vi "Import Asset Configuration.vi"(6 "Asset Configuration File":path, 8 "error in (no error)":errorcluster, 11 "InsightCM Console Wrapper in":refnum<class "InsightCM Console Wrapper.lvclass">) -> (0 "error out":errorcluster, 3 "InsightCM Console Wrapper out":refnum<class "InsightCM Console Wrapper.lvclass">)   [LabVIEW 2020, in "InsightCM Console Wrapper.lvclass"]
doc: "Imports asset configuration to the server using an Excel File (*.xlsx) exported form the same or another server.\n\nConsole command -> importassetspreadsheet -f [filepath]"
uses:
  InsightCM Console Wrapper.lvclass
  C:/Users/fflores/Documents/GitHub Projects/LabVIEW-CLI-Wrapper/Console Wrapper/Console Wrapper.lvclass
  Console Wrapper/Console Wrapper.lvclass/Console Wrapper.ctl
  Console Wrapper/Write Command Options.vi
  Console Wrapper/Write Command.vi
  Console Wrapper/Console Wrapper.lvclass
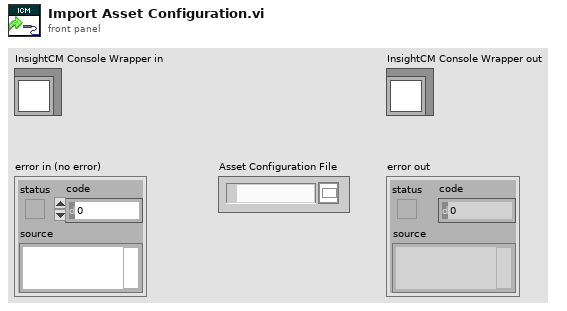
[diagram p1: front panel]
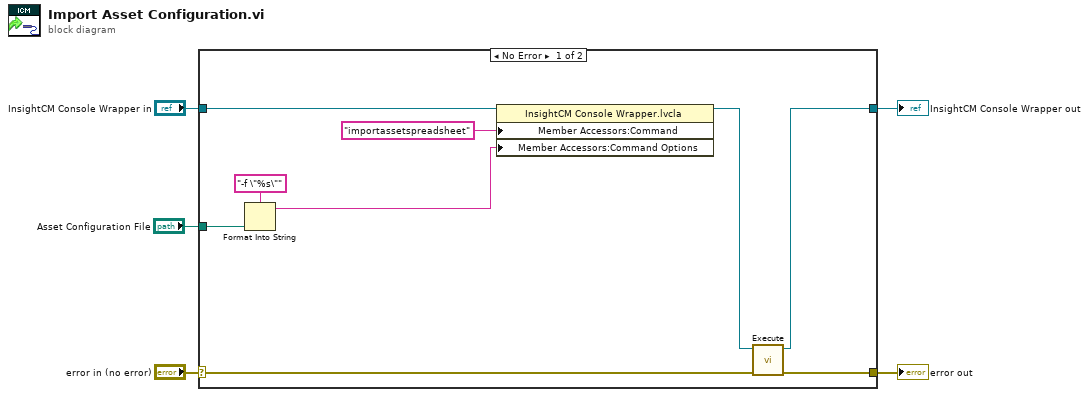
[diagram p0: block diagram]
diagram:
  n1 = case shown="No Error" "error in (no error)" {
    selector: "error in (no error)" -> [w14 w16]
    tunnel: [w13 w16] -> w4
    tunnel: [w11 w15] -> w2
    tunnel: "InsightCM Console Wrapper in" -> [w12 w15]
    tunnel: "Asset Configuration File" -> [w8 _]
    frame No Error {
      n2 = Format Into String(format string="-f \"%s\"", w8) -> (resulting string=w6:string)  [unwired: 2 in, 1 out]
      n3 = property class="InsightCM Console Wrapper.lvcla"(reference=w12, "Member Accessors:Command"="importassetspreadsheet" ("Command"), "Member Accessors:Command Options"=w6) -> (reference out=w10:refnum<class "InsightCM Console Wrapper.lvclass">)  [unwired: 1 in, 1 out]
      n4 = call "Execute.vi"("error in (no error)"=w14, "Console Wrapper in"=w10) -> ("error out"=w13:errorcluster, "Console Wrapper out"=w11:refnum<class "InsightCM Console Wrapper.lvclass">)  [unwired: 7 in, 1 out]
    }
    frame Error {
    }
  }
  "error out" <- w4
  "InsightCM Console Wrapper out" <- w2
